vi "Triangular Inverse CDF.vi"(8 "xmax":dbl=1.0, 9 "xmode":dbl=nan, 10 "xmin":dbl, 11 "cdf(x)":dbl=0.5) -> (0 "error":i32, 3 "x":dbl=0.5)   [LabVIEW 2018, in "NI_Gmath.lvlib"]
doc: "Computes the continuous inverse cumulative distribution function (CDF) of the various distributions. You must manually select the polymorphic instance to use."
uses:
  NI_Gmath.lvlib
  st_error_code.ctl
panel:
  # "Triangular Inverse CDF"
  # "NaN maps to \n(xmax-xmin)/2"
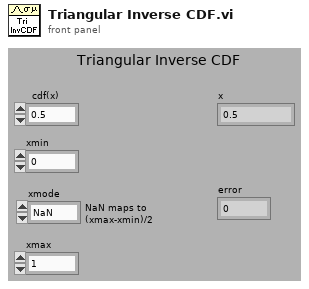
[diagram p1: front panel]
types:
  T1 = typedef "NI_Gmath.lvlib/st_error_code.ctl" = i32
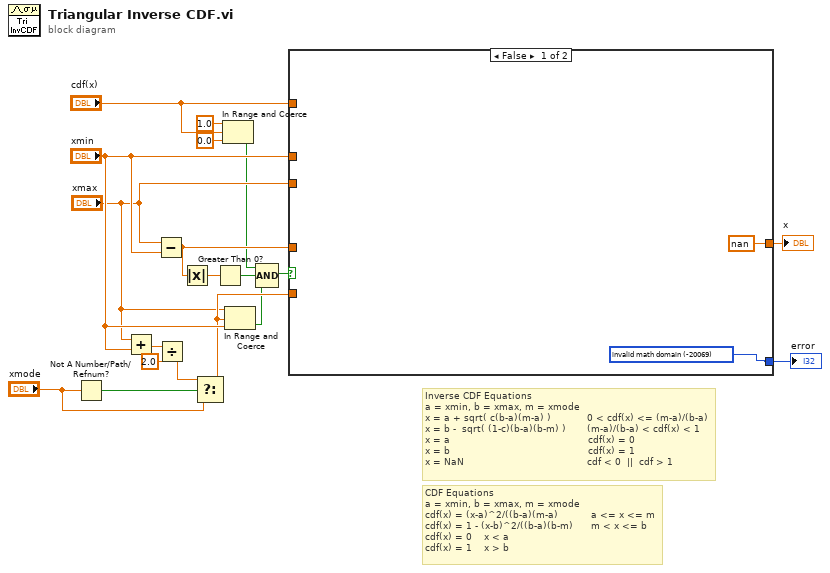
[diagram p0: block diagram]
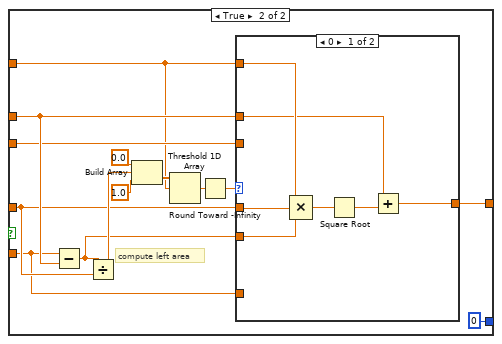
[diagram p2: hidden frame]
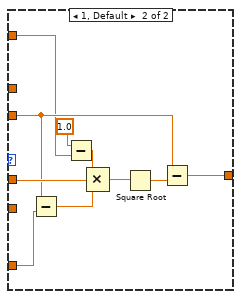
[diagram p3: hidden frame]
diagram:
  # "Inverse CDF Equations\na = xmin, b = xmax, m = xmode\nx = a + sqrt( c(b-a)(m-a) )            0 < cdf(x) <= (m-a)/(b-a)\nx = b -  sqrt( (1-c)(b-a)(b-m) )       (m-a)/(b-a) < cdf(x) < 1\nx = a                                              cdf(x) = 0\nx = b                                              cdf(x) = 1\nx = NaN                                         cdf < 0  ||  cdf > 1"
  # "CDF Equations\na = xmin, b = xmax, m = xmode\ncdf(x) = (x-a)^2/((b-a)(m-a)           a <= x <= m\ncdf(x) = 1 - (x-b)^2/((b-a)(b-m)      m < x <= b\ncdf(x) = 0    x < a\ncdf(x) = 1    x > b"
  n1 = Not A Number/Path/Refnum?(number/path/refnum="xmode") -> (NaN/Path/Refnum?=w11:bool)
  n2 = Add(x="xmax", y="xmin") -> (x+y=w14:dbl)
  n3 = Subtract(x="xmax", y="xmin") -> (x-y=w16:dbl)
  n4 = Divide(x=w14, y=2.0) -> (x/y=w12:dbl)
  n5 = Absolute Value(x=w16) -> (abs(x)=w19:dbl)
  n6 = Select(t=w12, s=w11, f="xmode") -> (s? t:f=w9:dbl)
  n7 = Greater Than 0?(x=w19) -> (x > 0?=w2:bool)
  n8 = In Range and Coerce(upper limit=1.0, x="cdf(x)", lower limit=0.0) -> (In Range?=w3:bool)  [unwired: 1 out]
  n9 = In Range and Coerce(upper limit="xmax", x=w9, lower limit="xmin") -> (In Range?=w1:bool)  [unwired: 1 out]
  n10 = Compound Arithmetic op=AND(w3, w2, w1) -> (w4:bool)
  n11 = case shown="False" w4 {
    tunnel: "cdf(x)" -> [_ w26]
    tunnel: "xmin" -> [_ w28]
    tunnel: w16 -> [_ w25]
    tunnel: [nan w23] -> w18
    tunnel: [w20 0] -> w17
    tunnel: w9 -> [_ w22]
    tunnel: "xmax" -> [_ w27]
    frame False {
      w20 = T1 -20069 items=["invalid math domain"=-20069, "Fourier interpolation size m >= n"=-20070, "empty array"=-20003] ("stat interp error code")
    }
    frame True {
      # "compute left area"
      n12 = Subtract(x=w22, y=w28) -> (x-y=w24:dbl)
      n13 = Divide(x=w24, y=w25) -> (x/y=w33:dbl)
      n14 = Build Array(0.0 ("element"), w33, 1.0 ("element")) -> (w31:dbl[])
      n15 = Threshold 1D Array(2:w26, 3:w31) -> (0:w30:dbl)  [unwired: 1 in]
      n16 = Round Toward -Infinity(1:w30) -> (0:w29:dbl)
      n17 = case shown="0" w29 {
        tunnel: w28 -> [w37 _]
        tunnel: w27 -> [_ w48]
        tunnel: w26 -> [w40 w44]
        tunnel: w25 -> [w41 w52]
        tunnel: w24 -> [w42 _]
        tunnel: [w36 w50] -> w23
        tunnel: w22 -> [_ w49]
        frame 0 {
          n18 = Compound Arithmetic op=MULTIPLY(w40, w41, w42) -> (w39:dbl)
          n19 = Square Root(x=w39) -> (sqrt(x)=w38:dbl)
          n20 = Add(x=w37, y=w38) -> (x+y=w36:dbl)
        }
        frame 1, Default {
          n21 = Subtract(x=w48, y=w49) -> (x-y=w47:dbl)
          n22 = Subtract(x=1.0 ("element"), y=w44) -> (x-y=w43:dbl)
          n23 = Compound Arithmetic op=MULTIPLY(w43, w52, w47) -> (w46:dbl)
          n24 = Square Root(x=w46) -> (sqrt(x)=w51:dbl)
          n25 = Subtract(x=w48, y=w51) -> (x-y=w50:dbl)
        }
      }
    }
  }
  "x" <- w18
  "error" <- w17
